vi "host_execute_command.vi"(8 "error in (no error)":errorcluster) -> (0 "error out":errorcluster)   [LabVIEW 2021]
uses:
  host_global_vars.vi
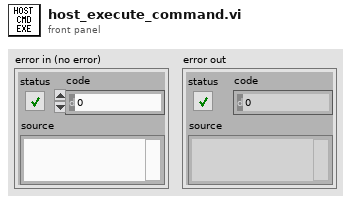
[diagram p1: front panel]
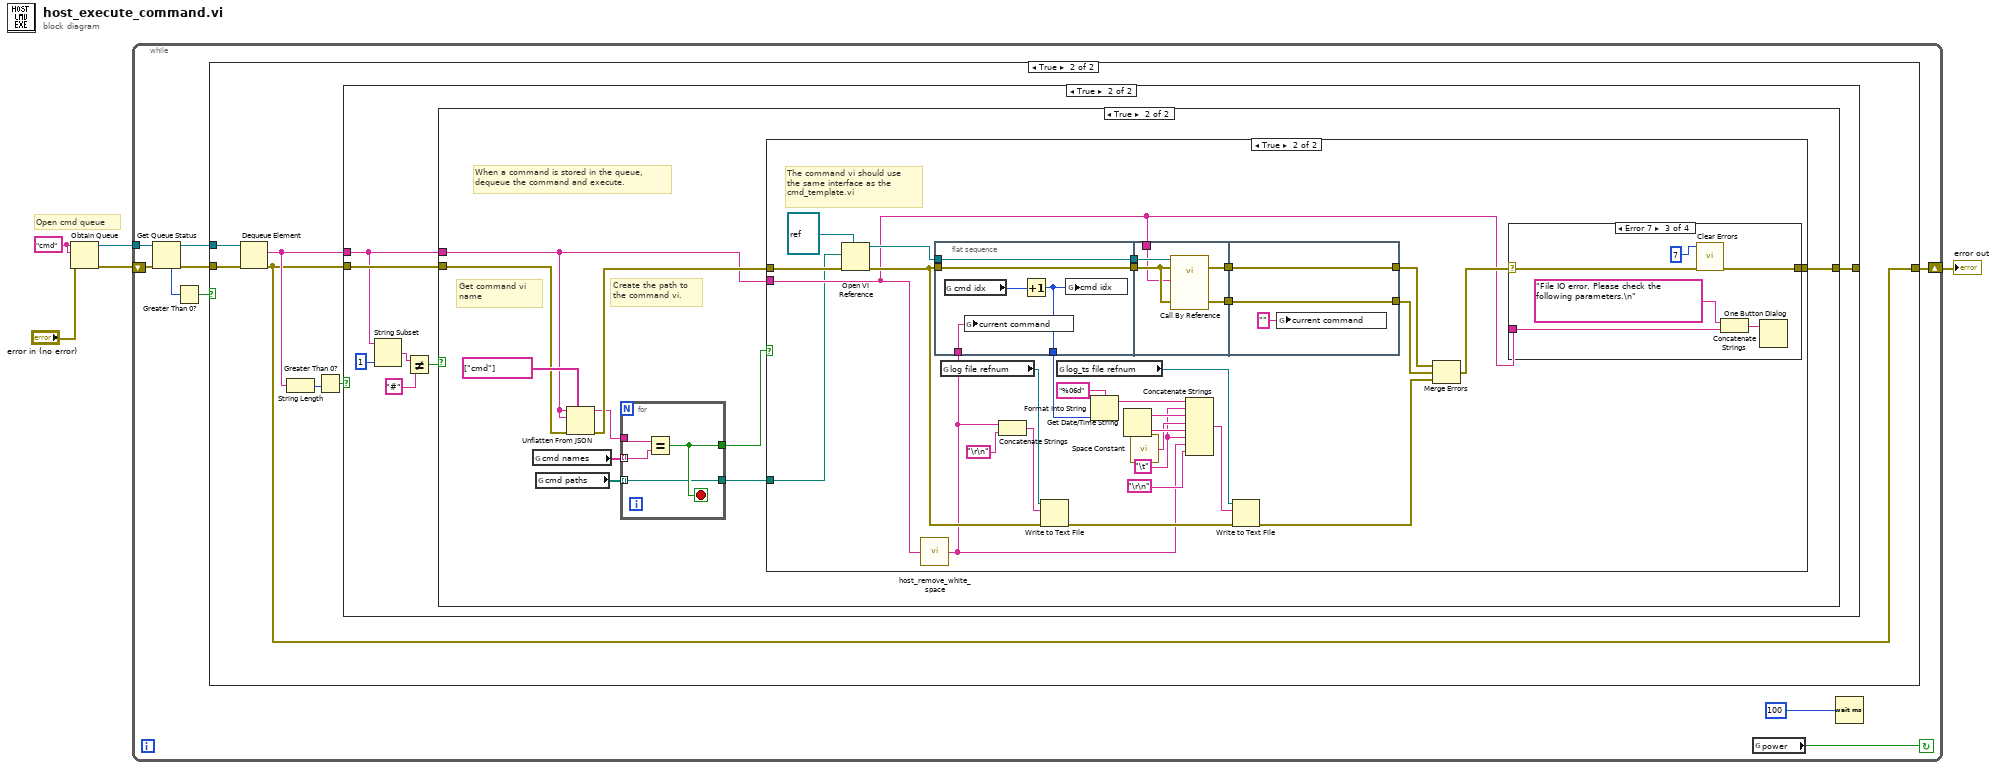
[diagram p0: block diagram]
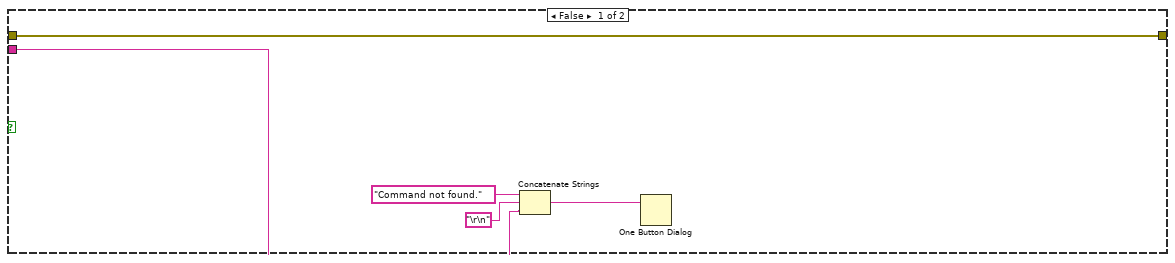
[diagram p5: hidden frame]
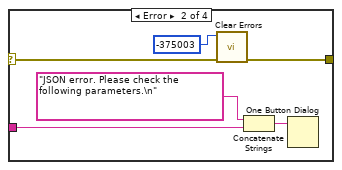
[diagram p7: hidden frame]
diagram:
  w4 = "cmd" ("name (unnamed)")
  # "Open cmd queue"
  n1 = Obtain Queue(name (unnamed)=w4, element data type=w4, error in (no error)="error in (no error)") -> (queue out=w2:refnum<queue>, error out=w3:errorcluster)  [unwired: 2 in, 1 out]
  n2 = while {
    tunnel: w2 -> [w13]
    shift-right: [w6] -> w1
    shift-left: w3 -> [w14]
    stop <- w8 continue-if-true
    n3 = Get Queue Status(queue=w13, error in (no error)=w14) -> (queue out=w10:refnum<queue>, error out=w9:errorcluster, # elements in queue=w12:i32)  [unwired: 1 in, 5 out]
    n4 = Greater Than 0?(x=w12) -> (x > 0?=w11:bool)
    n5 = case shown="True" w11 {
      tunnel: w10 -> [_ w21]
      tunnel: w9 -> [w15 w20]
      tunnel: [w15 w16] -> w6
      frame False {
      }
      frame True {
        n6 = Dequeue Element(queue=w21, error in (no error)=w20) -> (element=w17:string, error out=w16:errorcluster)  [unwired: 1 in, 2 out]
        n7 = String Length(string=w17) -> (length=w19:i32)
        n8 = Greater Than 0?(x=w19) -> (x > 0?=w18:bool)
        n9 = case shown="True" w18 {
          tunnel: w17 -> [_ w28]
          tunnel: [w22 w23] -> _
          tunnel: w16 -> [w22 w29]
          frame False {
          }
          frame True {
            n10 = String Subset(string=w28, length (rest)=1 ("length (rest)")) -> (substring=w26:string)  [unwired: 1 in]
            n11 = Not Equal?(x=w26, y="#") -> (x != y?=w24:bool)
            n12 = case shown="True" w24 {
              tunnel: [w30 w39] -> w23
              tunnel: w29 -> [w30 w38]
              tunnel: w28 -> [_ w31]
              frame False {
              }
              frame True {
                # "Create the path to \nthe command vi."
                # "Get command vi \nname"
                # "When a command is stored in the queue,\ndequeue the command and execute."
                n13 = global read "host_global_vars.vi" "cmd names"() -> (w36:string[])
                n14 = global read "host_global_vars.vi" "cmd paths"() -> (w35:path[])
                n15 = Unflatten From JSON(path=string[] ["cmd"], JSON string=w31, type and defaults=w31, error in (no error)=w38) -> (value=w34:string, error out=w37:errorcluster)  [unwired: 3 in]
                n16 = for {
                  tunnel: w36 -> [w105] mode=indexing
                  tunnel: w35 -> [w103] mode=indexing
                  tunnel: w34 -> [w106]
                  tunnel: [w104] -> w33
                  tunnel: [w103] -> w32
                  stop <- w104 stop-if-true
                  n17 = Equal?(x=w106, y=w105) -> (x = y?=w104:bool)
                }
                n18 = case shown="True" w33 {
                  tunnel: [w45 w67] -> w39
                  tunnel: w37 -> [w45 w66]
                  tunnel: w31 -> [w42 w48]
                  tunnel: w32 -> [_ w46]
                  frame False {
                    n19 = Concatenate Strings("Command not found." ("message"), "\r\n", w42) -> (w41:string)
                    n20 = One Button Dialog(message=w41) -> ()  [unwired: 1 in, 1 out]
                  }
                  frame True {
                    w52 = "\t"
                    # "The command vi should use\nthe same interface as the\ncmd_template.vi"
                    n21 = Open VI Reference(type specifier VI Refnum (for type only)=refnum<vi> refnum, vi path=w46, error in (no error)=w66) -> (vi reference=w69:refnum<vi>, error out=w70:errorcluster)  [unwired: 3 in]
                    n22 = call "host_remove_white_space.vi"("in"=w48) -> ("out"=w47:string)
                    n23 = flat-sequence {
                      tunnel: w70 -> [w79]
                      tunnel: w69 -> [w80]
                      tunnel: [w80] -> w75
                      tunnel: [w79] -> w74
                      tunnel: [w77] -> w50
                      tunnel: w47 -> [w76]
                      tunnel: w75 -> [w85]
                      tunnel: w74 -> [w84]
                      tunnel: w48 -> [w81]
                      tunnel: [w83] -> w73
                      tunnel: [w82] -> w72
                      tunnel: [w87] -> w53
                      tunnel: [w88] -> w54
                      tunnel: w73 -> [w88]
                      tunnel: w72 -> [w87]
                      frame #0 {
                        n24 = global read "host_global_vars.vi" "cmd idx"() -> (w78:i32)
                        n25 = global write "host_global_vars.vi" "current command"(w76) -> ()
                        n26 = Increment(x=w78) -> (x+1=w77:i32)
                        n27 = global write "host_global_vars.vi" "cmd idx"(w77) -> ()
                      }
                      frame #1 {
                        n28 = call-by-ref "?"(reference=w85, error in=w84, 8:"error in (no error)"=w84, "args"=w81) -> (error out=w82:errorcluster, 0:"error out"=w83:errorcluster)  [unwired: 9 in, 1 out]
                      }
                      frame #2 {
                        n29 = global write "host_global_vars.vi" "current command"("" ("current command")) -> ()
                      }
                    }
                    n30 = global read "host_global_vars.vi" "log file refnum"() -> (w65:refnum<file>)
                    n31 = Concatenate Strings(w47, "\r\n") -> (w59:string)
                    n32 = Write to Text File(file (use dialog)=w65, text=w59, error in=w70) -> (error out=w56:errorcluster)  [unwired: 1 in, 2 out]
                    n33 = global read "host_global_vars.vi" "log_ts file refnum"() -> (w57:refnum<file>)
                    n34 = Format Into String(format string="%06d", w50) -> (resulting string=w51:string)  [unwired: 2 in, 1 out]
                    n35 = Get Date/Time String() -> (date string=w64:string, time string=w63:string)  [unwired: 3 in]
                    n36 = call <vilib>:"Space Constant.vi"() -> ("String"=w62:string)
                    n37 = Concatenate Strings(w51, w52, w64, w62, w63, w52, w47, "\r\n") -> (w58:string)
                    n38 = Write to Text File(file (use dialog)=w57, text=w58, error in=w56) -> (error out=w55:errorcluster)  [unwired: 1 in, 2 out]
                    n39 = Merge Errors(w53, w54, w55) -> (w68:errorcluster)
                    n40 = case shown="Error 7" w68 {
                      selector: w68 -> [w89 w95 w101 w102]
                      tunnel: [w89 w94 w100 w102] -> w67
                      tunnel: w48 -> [_ w90 w96 _]
                      frame No Error {
                      }
                      frame Error {
                        n41 = call <vilib>:"Clear Errors.vi"("error in (no error)"=w95, "specific error code to clear (0: all)"=-375003) -> ("error out"=w94:errorcluster)  [unwired: 4 in, 1 out]
                        n42 = Concatenate Strings("JSON error. Please check the following parameters.\n", w90) -> (w91:string)
                        n43 = One Button Dialog(message=w91) -> ()  [unwired: 1 in, 1 out]
                      }
                      frame Error {
                        n44 = call <vilib>:"Clear Errors.vi"("error in (no error)"=w101, "specific error code to clear (0: all)"=7) -> ("error out"=w100:errorcluster)  [unwired: 4 in, 1 out]
                        n45 = Concatenate Strings("File IO error. Please check the following parameters.\n", w96) -> (w97:string)
                        n46 = One Button Dialog(message=w97) -> ()  [unwired: 1 in, 1 out]
                      }
                      frame Default {
                      }
                    }
                  }
                }
              }
            }
          }
        }
      }
    }
    n47 = global read "host_global_vars.vi" "power"() -> (w8:bool)
    n48 = Wait (ms)(milliseconds to wait=u32 100) -> ()  [unwired: 1 out]
  }
  "error out" <- w1
